vi "6_ВППереводТемпературы.vi"() -> ()   [LabVIEW 2016]
panel:
  out "Град F":dbl
  in  "Град С":dbl
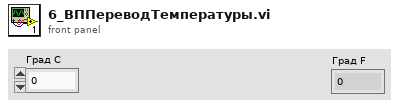
[diagram p1: front panel]
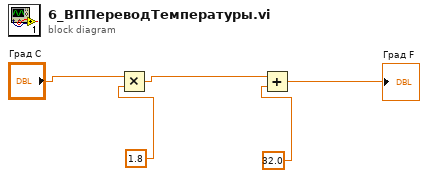
[diagram p0: block diagram]
diagram:
  n1 = Multiply(x="Град С", y=1.8) -> (x*y=w3:dbl)
  n2 = Add(x=w3, y=32.0) -> (x+y=→"Град F":dbl)
